vi "main-tempToImgForMovie.vi"() -> ()   [LabVIEW 2009]
panel:
  out "Postęp":string
  out "Proces przetwarzania zdjęć":u8(slide) scale=0.0..100.0
  out "temp dla wybranego kanału":i32
  out "naglowek":i32
  out "godzina z temp":i32
  out "godzina zdjecia":i32
  out "lista zdjec":i32
  out "fps":i32
  out "Nr zdjecia":i32
  out "rainbow size":i32
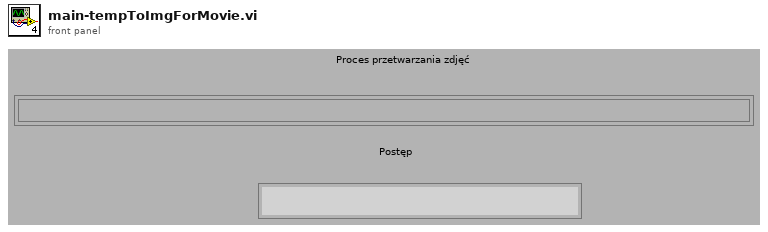
[diagram p1: front panel]
types:
  T1 = cluster{"Left":i32, "Top":i32, "Right":i32, "Bottom":i32}
  T2 = typedef "IMAQ Image.ctl" = refnum<image>
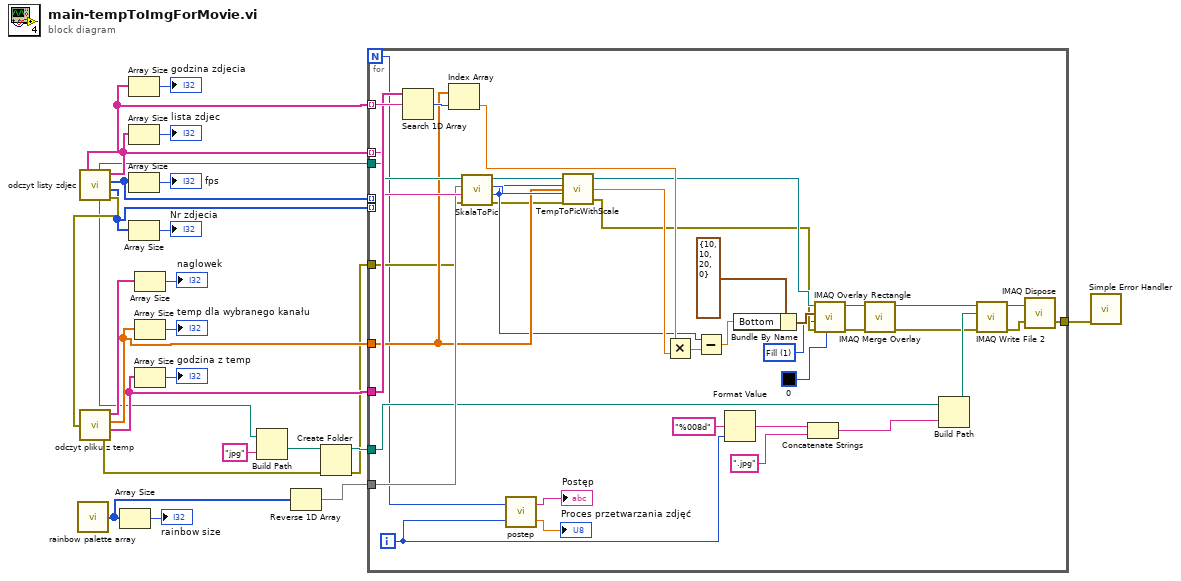
[diagram p0: block diagram]
diagram:
  n1 = call "rainbow palette array.vi"() -> ("rainbow array"=w9:u32[])  [unwired: 1 in]
  n2 = call "odczyt listy zdjec.vi"() -> ("error out"=w16:errorcluster, "Nr zdjecia"=w12:i32[], "fps"=w13:i32[], "lista zdjec"=w14:string[], "sciezka do zdjec"=w4:path, "godzina ze zdjecia"=w15:string[])  [unwired: 1 in]
  n3 = call "odczyt pliku z temp.vi"("error in (no error)"=w16) -> ("Nagłówki (tablica 1D)"=w18:string[], "Temperatury (wybrany kanał)"=w11:dbl[], "Kolumna z czasem (tablica 1D)"=w10:string[], "error out"=w7:errorcluster)
  n4 = Array Size(array=w9) -> (size(s)=→"rainbow size":i32)
  n5 = Array Size(array=w15) -> (size(s)=→"godzina zdjecia":i32)
  n6 = Array Size(array=w14) -> (size(s)=→"lista zdjec":i32)
  n7 = Array Size(array=w13) -> (size(s)=→"fps":i32)
  n8 = Array Size(array=w12) -> (size(s)=→"Nr zdjecia":i32)
  n9 = Array Size(array=w18) -> (size(s)=→"naglowek":i32)
  n10 = Array Size(array=w11) -> (size(s)=→"temp dla wybranego kanału":i32)
  n11 = Array Size(array=w10) -> (size(s)=→"godzina z temp":i32)
  n12 = Build Path(base path=w4, name or relative path="jpg") -> (appended path=w3:path)
  n13 = Reverse 1D Array(array=w9) -> (reversed array=w1:u32[])
  n14 = Create Folder(path (use dialog)=w3, error in=w7) -> (created path=w8:path, error out=w6:errorcluster)  [unwired: 1 in, 1 out]
  n15 = for {
    N -> [w28]
    tunnel: w15 -> [w64] mode=indexing
    tunnel: w14 -> [w59] mode=indexing
    tunnel: w13 -> [_] mode=indexing
    tunnel: w12 -> [_] mode=indexing
    tunnel: w11 -> [w55]
    tunnel: w10 -> [w63]
    tunnel: w1 -> [w58]
    tunnel: w4 -> [w60]
    tunnel: w8 -> [w46]
    tunnel: w6 -> [w40]
    tunnel: [w26] -> w5
    i -> [w29]
    w38 = u32 1 items=["Frame", "Fill", "Highlight"] ("Drawing Mode (Frame)")
    n16 = Search 1D Array(1D array=w63, element=w64) -> (index of element=w62:i32)  [unwired: 1 in]
    n17 = Index Array(array=w55, index=w62) -> (element=w54:dbl)
    n18 = call "SkalaToPic.vi"("error in (no error)"=w40, "nazwa pliku zdjęcia"=w59, "rainbow array"=w58, "Katalog z plikami"=w60) -> ("error out"=w41:errorcluster, "Bottom prost."=w48:i32, "rozdzielczość obrazu pomniejszona o 30px"=w56:i32, "Image Out"=w57:T2)
    n19 = call "postep.vi"("kolejne powtórzenie pętli"=w29, "Całość do przetworzenia"=w28) -> ("Proces przetwarzania zdjęć"=→"Proces przetwarzania zdjęć":dbl, "Postęp"=→"Postęp":string)
    n20 = call "TempToPicWithScale.vi"("Image with Scale"=w57, "Bottom prost."=w48, "rozdzielczość obrazu pomniejszona o 30px"=w56, "error in (no error)"=w41, "Temperatury (wybrany kanał)"=w55) -> ("Image Out"=w52:T2, "step dla 1stC"=w53:dbl, "error out"=w42:errorcluster)
    n21 = Multiply(x=w54, y=w53) -> (x*y=w47:dbl)
    n22 = Subtract(x=w48, y=w47) -> (x-y=w33:dbl)
    n23 = Format Value(format string="%008d", value (0)=w29) -> (output string=w31:string)  [unwired: 1 in]
    n24 = Bundle By Name(cluster=T1 {"Left"=10, "Top"=10, "Right"=20, "Bottom"=0} ("Rectangle"), "Bottom"=w33) -> (w50:T1)
    n25 = Concatenate Strings(w31, ".jpg" ("string")) -> (w45:string)
    n26 = call "IMAQ Overlay Rectangle"("Color"=u32 0, "error in (no error)"=w42, "Drawing Mode (Frame)"=w38, "Rectangle"=w50, "Image"=w52) -> ("error out"=w36:errorcluster, "Image Out"=w34:T2)  [unwired: 5 in]
    n27 = call "IMAQ Merge Overlay"("error in (no error)"=w36, "Image Src"=w34) -> ("error out"=w35:errorcluster, "Image Dst Out"=w37:T2)  [unwired: 8 in]
    n28 = Build Path(base path=w46, name or relative path=w45) -> (appended path=w43:path)
    n29 = call-poly "IMAQ Write File 2"("error in (no error)"=w35, "File Path"=w43, "Image"=w37) -> ("error out"=w27:errorcluster, "Image Out (duplicate)"=w39:T2)  [unwired: 7 in]
    n30 = call "IMAQ Dispose"("Image"=w39, "error in (no error)"=w27) -> ("error out"=w26:errorcluster)  [unwired: 4 in]
  }
  n31 = call <vilib>:"Simple Error Handler.vi"("error in (no error)"=w5) -> ()  [unwired: 4 in, 5 out]
